vi "FTW-Connector-SpawnNewActor.vi"(0 "FTW Actor Connector Type":refnum<class "FTW-ActorConnector.lvclass">, 5 "Configuration":string="{\n  \"Identity\": \"ActorName\",\n  \"DebugEnableInboxLogging\": false,\n  \"DebugEnableJobLogging\": false,\n  \"InboxAddress\": \"inproc://*\",\n  \"PublisherAddress\": \"lvn://*\",\n  \"DebugShowPanel\": false\n}", 7 "Actor VI Filepath":path, 9 "Timeout":i32=1000 format="%dmsec", 11 "error in":errorcluster) -> (4 "FTW Actor Connector":refnum<class "FTW-ActorConnector.lvclass">, 6 "Initialized Response":string, 8 "Instance Inbox Address":string, 10 "Deprecated":string, 15 "error out":errorcluster)   [LabVIEW 2013, in "FTW-ActorConnector.lvclass"]
uses:
  FTW-ActorConnector.lvclass
  Endpoint/FTW-Endpoint.lvclass
  Ether/FTW-Ether.lvclass
panel:
  # "Inputs"
  # "Outputs"
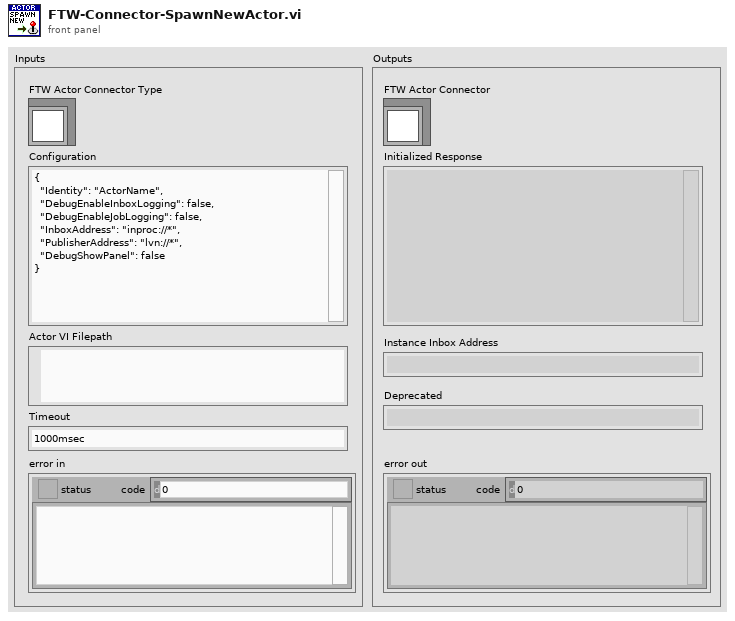
[diagram p1: front panel]
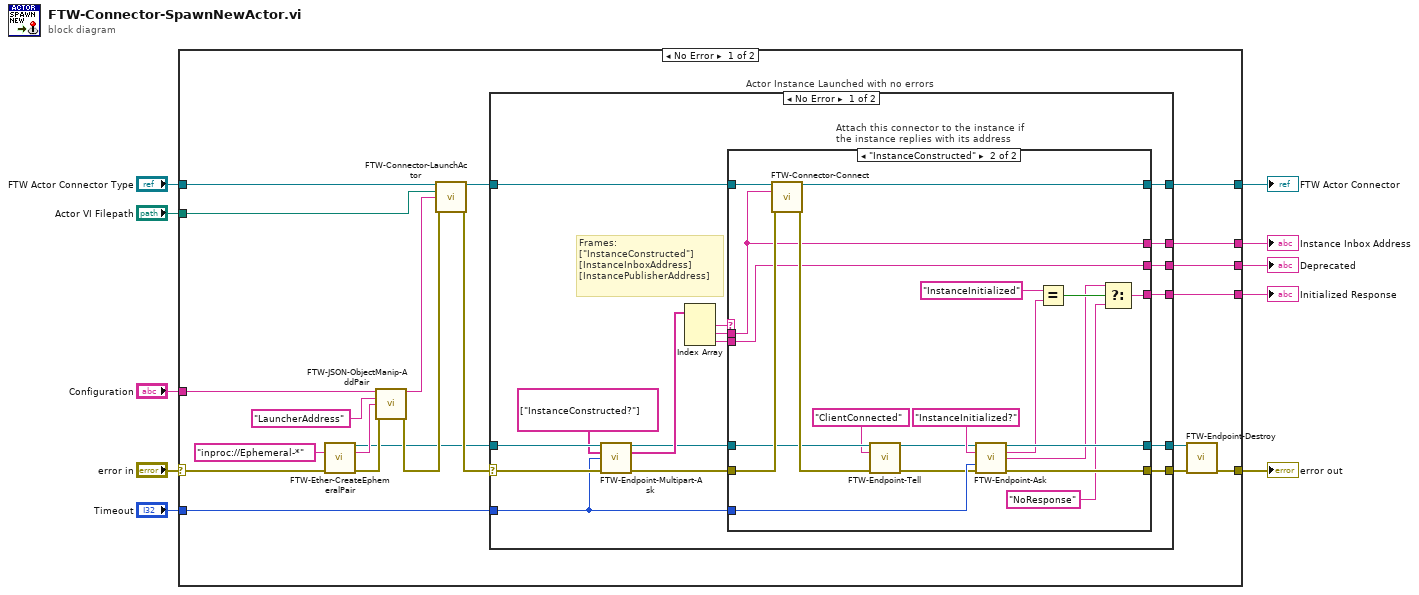
[diagram p0: block diagram]
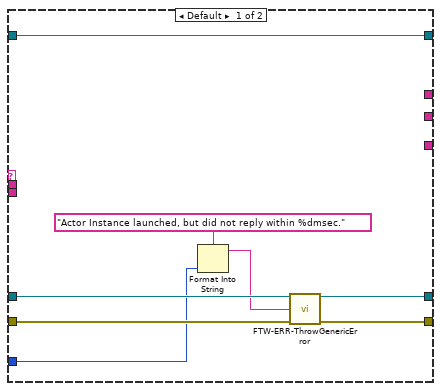
[diagram p2: hidden frame]
diagram:
  n1 = case shown="No Error" "error in" {
    selector: "error in" -> [w28 w80]
    tunnel: [w24 w80] -> w5
    tunnel: [w31 w79] -> w6
    tunnel: "FTW Actor Connector Type" -> [w23 w79]
    tunnel: "Configuration" -> [w30 _]
    tunnel: "Timeout" -> [w27 _]
    tunnel: "Actor VI Filepath" -> [w14 _]
    tunnel: [w19 _] -> w3
    tunnel: [w18 _] -> w2
    tunnel: [w17 _] -> w1
    frame No Error {
      n2 = call "FTW-Ether-CreateEphemeralPair.vi"("Requested Ephemeral Address"="inproc://Ephemeral-*", "error in"=w28) -> ("Ephemeral Endpoint"=w11:refnum<class "FTW-Endpoint.lvclass">, "Actual Ephemeral Address"=w16:string, "error out"=w15:errorcluster)  [unwired: 11 in]
      n3 = call "FTW-JSON-ObjectManip-AddPair.vi"("Input JSON Object"=w30, "Key"="LauncherAddress", "Value"=w16, "error in"=w15) -> ("Output JSON Object"=w13:string, "error out"=w21:errorcluster)  [unwired: 10 in]
      n4 = call-dynamic "FTW-Connector-LaunchActor.vi"("FTW Actor Connector Type"=w23, "Actor VI Filepath"=w14, "Configuration"=w13, "error in"=w21) -> ("FTW Actor Connector"=w22:refnum<class "FTW-ActorConnector.lvclass">, "error out"=w20:errorcluster)  [unwired: 10 in]
      n5 = case "Actor Instance Launched with no errors" shown="No Error" w20 {
        selector: w20 -> [w40 w77]
        tunnel: [w48 w77] -> w25
        tunnel: w22 -> [w47 w78]
        tunnel: [w46 w78] -> w31
        tunnel: w11 -> [w41 w76]
        tunnel: w27 -> [w39 _]
        tunnel: [w45 w76] -> w26
        tunnel: [w34 _] -> w19
        tunnel: [w33 _] -> w18
        tunnel: [w32 _] -> w17
        frame No Error {
          # "Frames:\n[\"InstanceConstructed\"]\n[InstanceInboxAddress]\n[InstancePublisherAddress]"
          n6 = call-dynamic "FTW-Endpoint-Multipart-Ask.vi"("FTW Endpoint"=w41, "Multipart Message"=string[] ["InstanceConstructed?"], "Read Timeout"=w39, "error in"=w40) -> ("FTW Endpoint out"=w35:refnum<class "FTW-Endpoint.lvclass">, "Reply"=w37:string[], "error out"=w36:errorcluster)  [unwired: 7 in, 2 out]
          n7 = Index Array(array=w37) -> (element #1=w44:string, element #2=w43:string, element #3=w42:string)  [unwired: 3 in]
          n8 = case "Attach this connector to the instance if\nthe instance replies with its address" shown="\"InstanceConstructed\"" w44 {
            tunnel: [w53 w70] -> w48
            tunnel: w47 -> [w55 w73]
            tunnel: [w55 w72] -> w46
            tunnel: w35 -> [w52 w59]
            tunnel: w36 -> [w54 w74]
            tunnel: [w52 w71] -> w45
            tunnel: w39 -> [w50 w62]
            tunnel: w43 -> [_ w60]
            tunnel: w42 -> [_ w61]
            tunnel: [_ w63] -> w34
            tunnel: [_ w61] -> w33
            tunnel: [_ w60] -> w32
            frame Default {
              n9 = Format Into String(format string="Actor Instance launched, but did not reply within %dmsec." ("Error Message"), w50) -> (resulting string=w49:string)  [unwired: 2 in, 1 out]
              n10 = call "FTW-ERR-ThrowGenericError.vi"("Error Message"=w49, "error in"=w54) -> ("error out"=w53:errorcluster)  [unwired: 13 in]
            }
            frame "InstanceConstructed" {
              n11 = call-dynamic "FTW-Connector-Connect.vi"("FTW Actor Connector Type"=w73, "Instance Inbox Address"=w60, "error in"=w74) -> ("FTW Actor Connector"=w72:refnum<class "FTW-ActorConnector.lvclass">, "error out"=w75:errorcluster)  [unwired: 11 in]
              n12 = call-dynamic "FTW-Endpoint-Tell.vi"("FTW Endpoint"=w59, "Message Header"="ClientConnected", "error in"=w75) -> ("FTW Endpoint out"=w58:refnum<class "FTW-Endpoint.lvclass">, "error out"=w57:errorcluster)  [unwired: 10 in, 1 out]
              n13 = call-dynamic "FTW-Endpoint-Ask.vi"("FTW Endpoint"=w58, "Request Header"="InstanceInitialized?", "Timeout"=w62, "error in"=w57) -> ("FTW Endpoint out"=w71:refnum<class "FTW-Endpoint.lvclass">, "Response Header"=w67:string, "Response Body"=w65:string, "error out"=w70:errorcluster)  [unwired: 6 in, 2 out]
              n14 = Equal?(x="InstanceInitialized", y=w67) -> (x = y?=w66:bool)
              n15 = Select(t=w65, s=w66, f="NoResponse") -> (s? t:f=w63:string)
            }
          }
        }
        frame Error {
        }
      }
      n16 = call-dynamic "FTW-Endpoint-Destroy.vi"("FTW Endpoint"=w26, "error in"=w25) -> ("error out"=w24:errorcluster)  [unwired: 13 in]
    }
    frame Error {
    }
  }
  "error out" <- w5
  "FTW Actor Connector" <- w6
  "Initialized Response" <- w3
  "Instance Inbox Address" <- w1
  "Deprecated" <- w2
